vi "Configure Trigger (Pulse).vi"(0 "VISA resource name":refnum<visa-resource-name>, 1 "Pulse Width (0.00)":dbl format="%_3g", 5 "Trigger Source (0: Channel 1)":i32(ring) items=["Channel 1", "Channel 2", "Channel 3", "Channel 4", "External Input", "Attenuated External Input"], 7 "Trigger Level (0.0 V)":dbl format="%_3g", 9 "Trigger Mode (0: Auto)":i32(ring) items=["Auto", "Normal"], 11 "error in (no error)":errorcluster, 12 "Holdoff (0.00)":dbl format="%_3g", 13 "Polarity (0: Positive)":i32(ring) items=["Positive", "Negative"], 14 "Trigger Condition (0: Equal)":i32(ring) items=["Equal", "Not Equal", "Inside", "Outside"]) -> (4 "VISA resource out":refnum<visa-resource-name>, 15 "error out":errorcluster)   [LabVIEW 2015, in "Tektronix TDS 200 1000 2000 Series.lvlib"]
doc: "Sets triggering to pulse mode, and configures the trigger options.\n\n<B>Note(s):</B>\nAvailable on TDS 1000 and 2000 series only."
uses:
  <instrlib>/Tektronix TDS 200 1000 2000 Series/Tektronix TDS 200 1000 2000 Series.lvlib
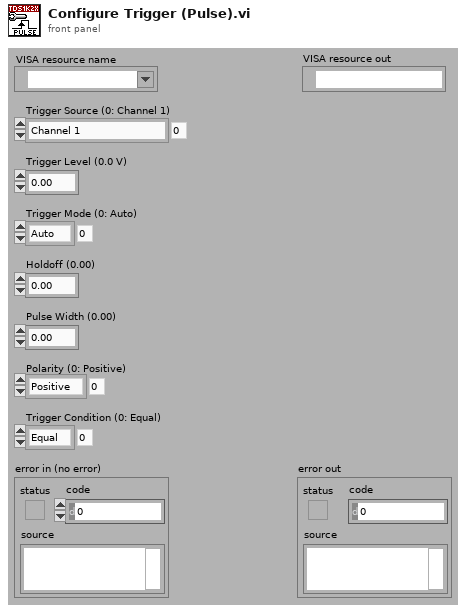
[diagram p1: front panel]
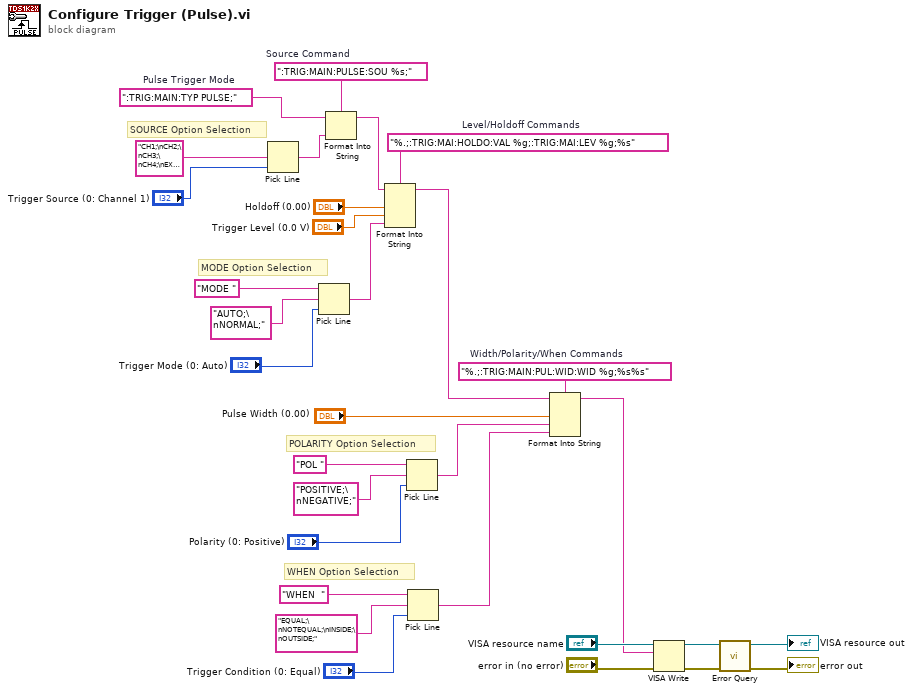
[diagram p0: block diagram]
diagram:
  w26 = "%.;:TRIG:MAIN:PUL:WID:WID %g;%s%s"  # Width/Polarity/When Commands
  w28 = "%.;:TRIG:MAI:HOLDO:VAL %g;:TRIG:MAI:LEV %g;%s"  # Level/Holdoff Commands
  w31 = ":TRIG:MAIN:TYP PULSE;"  # Pulse Trigger Mode
  w30 = ":TRIG:MAIN:PULSE:SOU %s;"  # Source Command
  # "MODE Option Selection"
  # "SOURCE Option Selection"
  # "WHEN Option Selection"
  # "POLARITY Option Selection"
  n1 = Pick Line(multi-line string="CH1;\nCH2;\nCH3;\nCH4;\nEXT;\nEXT5;", line index="Trigger Source (0: Channel 1)") -> (output string=w7:string)  [unwired: 1 out]
  n2 = Pick Line(string ("")="MODE ", multi-line string="AUTO;\nNORMAL;", line index="Trigger Mode (0: Auto)") -> (output string=w1:string)
  n3 = Format Into String(format string=w30, initial string=w31, w7) -> (resulting string=w29:string)  [unwired: 1 in, 1 out]
  n4 = Format Into String(format string=w28, initial string=w29, "Holdoff (0.00)", "Trigger Level (0.0 V)", w1) -> (resulting string=w25:string)  [unwired: 1 in, 1 out]
  n5 = Pick Line(string ("")="POL ", multi-line string="POSITIVE;\nNEGATIVE;", line index="Polarity (0: Positive)") -> (output string=w16:string)
  n6 = Pick Line(string ("")="WHEN  ", multi-line string="EQUAL;\nNOTEQUAL;\nINSIDE;\nOUTSIDE;", line index="Trigger Condition (0: Equal)") -> (output string=w11:string)
  n7 = Format Into String(format string=w26, initial string=w25, "Pulse Width (0.00)", w16, w11) -> (resulting string=w10:string)  [unwired: 1 in, 1 out]
  n8 = VISA Write(VISA resource name="VISA resource name", write buffer=w10, error in (no error)="error in (no error)") -> (VISA resource name out=w20:refnum<visa-resource-name>, error out=w18:errorcluster)  [unwired: 1 out]
  n9 = call <instrlib>:"Error Query.vi"("error in (no error)"=w18, "VISA resource name"=w20) -> ("error out"=→"error out":errorcluster, "VISA resource name out"=→"VISA resource out":refnum<visa-resource-name>)  [unwired: 8 out]
